vi "parse.vi"(8 "error in (no error)":errorcluster, 10 "Frame":T1 {"Data" format="%02x"}, 11 "FrameParser in":refnum<class "FrameParser.lvclass">) -> (0 "error out":errorcluster, 3 "FrameParser out":refnum<class "FrameParser.lvclass">)   [LabVIEW 2015, in "RTModbus.lvlib" / "FrameParser.lvclass"]
uses:
  FrameParser.lvclass
  DataTypes/Frame.ctl
  FrameParser.lvclass/FrameParser.ctl
  RTModbus.lvlib
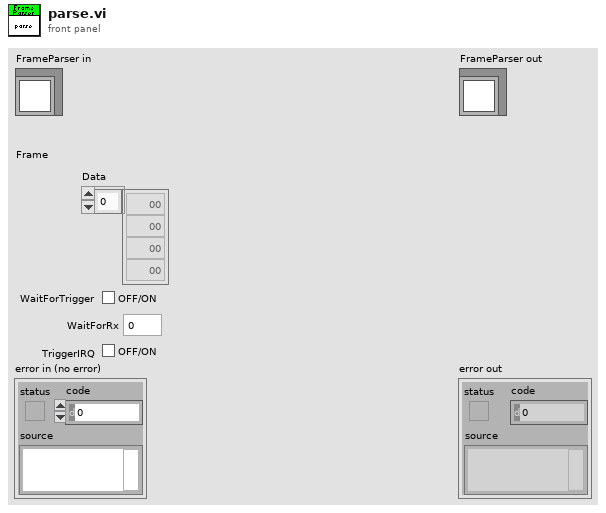
[diagram p1: front panel]
types:
  T1 = typedef "RTModbus.lvlib/Frame.ctl" = cluster{"Data":u8[], "WaitForTrigger":bool, "WaitForRx":u16, "TriggerIRQ":bool}
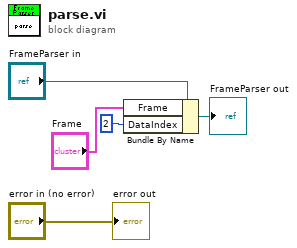
[diagram p0: block diagram]
diagram:
  n1 = Bundle By Name(cluster="FrameParser in", "Frame"="Frame", "DataIndex"=2) -> (→"FrameParser out":refnum<class "FrameParser.lvclass">)
  "error out" <- "error in (no error)"
